vi "Find_GT_File_Path.vi"(10 "GT Mask Folder Path":path=path "D:/DNN/MVTec/pill/ground_truth", 11 "Image File Path":path=path "D:/DNN/MVTec/pill/ground_truth") -> (2 "GT File Path":path, 3 "Image File Path out":path=path "D:/DNN/MVTec/pill/ground_truth")   [LabVIEW 2020]
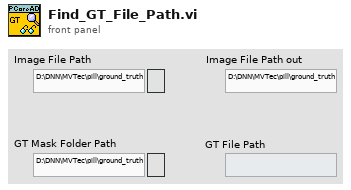
[diagram p1: front panel]
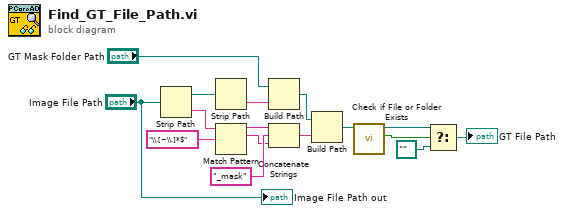
[diagram p0: block diagram]
diagram:
  n1 = Strip Path(path="Image File Path") -> (stripped path=w16:path, name=w9:string)
  n2 = Strip Path(path=w16) -> (name=w15:string)  [unwired: 1 out]
  n3 = Match Pattern(string=w9, regular expression="\\.[~\\.]*$") -> (before substring=w7:string, match substring=w6:string)  [unwired: 3 out]
  n4 = Build Path(base path="GT Mask Folder Path", name or relative path=w15) -> (appended path=w14:path)
  n5 = Concatenate Strings(w7, "_mask" ("string"), w6) -> (w13:string)
  n6 = Build Path(base path=w14, name or relative path=w13) -> (appended path=w10:path)
  n7 = call <vilib>:"Check if File or Folder Exists.vi"("path"=w10) -> ("file or folder exists?"=w5:bool, "dup path"=w4:path)  [unwired: 8 in, 1 out]
  n8 = Select(t=w4, s=w5, f=path "") -> (s? t:f=→"GT File Path":path)
  "Image File Path out" <- "Image File Path"
